vi "ClimbGetSensorPoseLeft.vi"() -> (1 "ClimbGetSensorPoseLeft":dbl)   [LabVIEW 2023]
uses:
  ClimbGlobal.vi
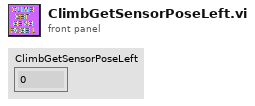
[diagram p1: front panel]
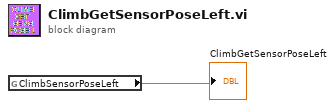
[diagram p0: block diagram]
diagram:
  n1 = global read "ClimbGlobal.vi" "ClimbSensorPoseLeft"() -> (→"ClimbGetSensorPoseLeft":dbl)
